vi "DAC Run.vi"(8 "error in":errorcluster, 11 "DAC Heater Box Temperatures in":refnum<class "DAC Heater Box Temperatures.lvclass">) -> (0 "error out":errorcluster, 3 "DAC Heater Box Temperatures out":refnum<class "DAC Heater Box Temperatures.lvclass">)   [LabVIEW 2019, in "DAC.lvlib" / "DAC Heater Box Temperatures.lvclass"]
uses:
  DAC Heater Box Temperatures.lvclass
  C:/Users/krio/Documents/LV_Projects/TestStand/App/DAC/DAC.lvclass
  DAC.lvclass/DAC.ctl
  Results/LNG Boiling Results/LNG Boiling Results.lvclass
  Results/Results Method.ctl
  DAC Heater Box Temperatures.lvclass/DAC Heater Box Temperatures.ctl
  <vilib>/DAQmx/read.llb/DAQmx Read (Analog 1D Wfm NChan 1Samp).vi
  <vilib>/DAQmx/miscellaneous.llb/DAQmx Fill In Error Info.vi
  DAC.lvclass
  Results/Results.lvlib
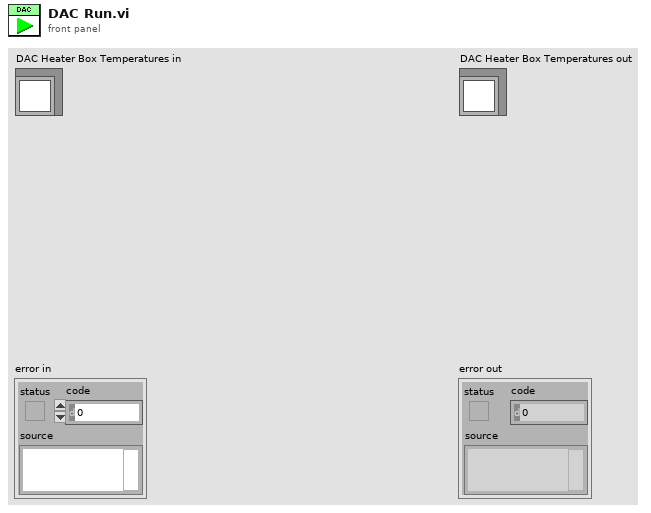
[diagram p1: front panel]
types:
  T1 = typedef "Results.lvlib/Results Method.ctl" = enum16{"Get", "Set"}
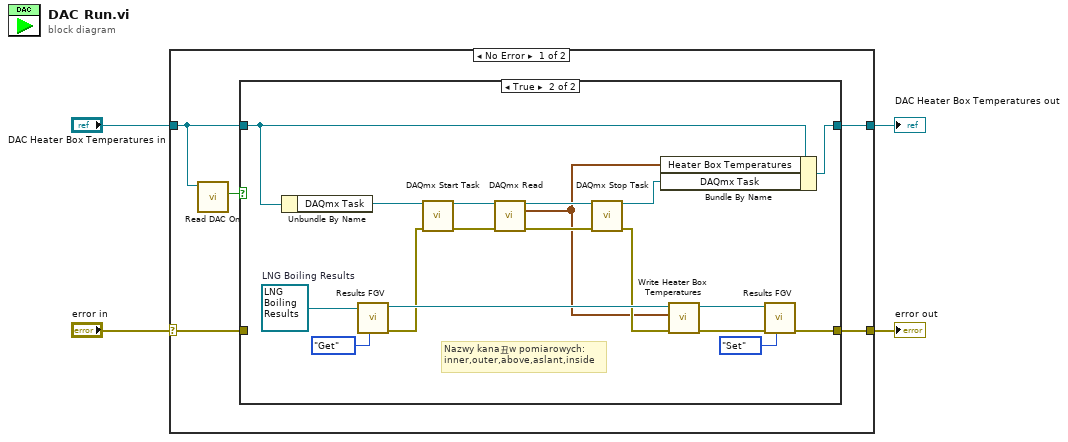
[diagram p0: block diagram]
diagram:
  n1 = case shown="No Error" "error in" {
    selector: "error in" -> [w7 w31]
    tunnel: [w6 w31] -> w2
    tunnel: [w8 w30] -> w1
    tunnel: "DAC Heater Box Temperatures in" -> [w5 w30]
    frame No Error {
      n2 = call "Read DAC On.vi"("DAC in"=w5) -> ("DAC On"=w9:bool)  [unwired: 8 in, 2 out]
      n3 = case shown="True" w9 {
        tunnel: w5 -> [w11 w24]
        tunnel: [w11 w15] -> w8
        tunnel: w7 -> [w10 _]
        tunnel: [w10 w14] -> w6
        frame False {
        }
        frame True {
          w23 = refnum<class "LNG Boiling Results.lvclass"> refnum  # LNG Boiling Results
          # "Nazwy kana丑w pomiarowych:\ninner,outer,above,aslant,inside"
          n4 = Unbundle By Name(w24) -> ("DAQmx Task"=w29:refnum<k21>)
          n5 = call-dynamic "Results FGV.vi"("Method"=Results_Method."Get", "LNG Boiling Results in"=w23) -> ("error out"=w18:errorcluster, "LNG Boiling Results out"=w22:refnum<class "LNG Boiling Results.lvclass">)  [unwired: 8 in]
          n6 = call <vilib>:"DAQmx Start Task.vi"("task/channels in"=w29, "error in"=w18) -> ("task out"=w28:refnum<k21>, "error out"=w26:errorcluster)  [unwired: 12 in]
          n7 = call-poly <vilib>:"DAQmx Read.vi"("task/channels in"=w28, "error in"=w26) -> ("task out"=w27:refnum<k21>, "data"=w12:waveform(dbl)[], "error out"=w25:errorcluster)  [unwired: 11 in]
          n8 = call <vilib>:"DAQmx Stop Task.vi"("task/channels in"=w27, "error in"=w25) -> ("task out"=w13:refnum<k21>, "error out"=w17:errorcluster)  [unwired: 12 in]
          n9 = Bundle By Name(cluster=w24, "Heater Box Temperatures"=w12, "DAQmx Task"=w13) -> (w15:refnum<class "DAC Heater Box Temperatures.lvclass">)
          n10 = call-dynamic "Write Heater Box Temperatures.vi"("error in (no error)"=w17, "Heater Box Temperatures"=w12, "LNG Boiling Results in"=w22) -> ("error out"=w16:errorcluster, "LNG Boiling Results out"=w21:refnum<class "LNG Boiling Results.lvclass">)  [unwired: 7 in]
          n11 = call-dynamic "Results FGV.vi"("Method"=Results_Method."Set", "error in"=w16, "LNG Boiling Results in"=w21) -> ("error out"=w14:errorcluster)  [unwired: 7 in, 1 out]
        }
      }
    }
    frame Error {
    }
  }
  "error out" <- w2
  "DAC Heater Box Temperatures out" <- w1
